vi "ConfigureMeasurementParameters.vi"(0 "NI-DMM in":refnum<class "NI-DMM.lvclass">, 5 "Configure_Parameters":variant, 11 "error in (no error)":errorcluster) -> (4 "NI-DMM out":refnum<class "NI-DMM.lvclass">, 15 "error out":errorcluster)   [LabVIEW 2020, in "Abstract_Instrument.lvlib" / "NI-DMM.lvclass"]
uses:
  NI-DMM.lvclass
  TypeDef/Configure_Parameters.ctl
  <instrlib>/niDMM/nidmm.llb/niDMM Resolution in Digits.ctl
  <instrlib>/niDMM/nidmm.llb/niDMM Configure Measurement Digits.vi
  <vilib>/MeasurementLink/MeasurementLink niDMM/MeasurementLink niDMM.lvlib
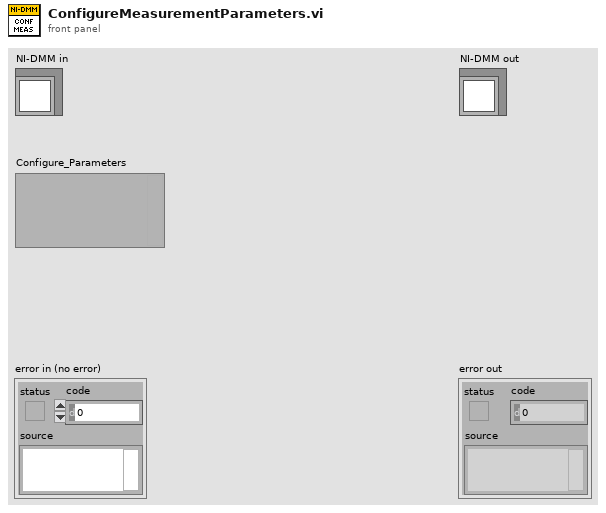
[diagram p1: front panel]
types:
  T1 = typedef "Abstract_Instrument.lvlib/NI-DMM.lvclass/Configure_Parameters.ctl" = cluster{"Range":dbl, "Measurement Type":enum32{"DC Volts", "AC Volts", "DC Current", "AC Current", "2-wire Resistance", "4-wire Resistance", "Diode", "Frequency", "Period", "AC Volts DC Coupled", "Capacitance", "Inductance", "Temperature"}, "Resolution in Digits":enum32{"3 1/2", "4 1/2", "5 1/2", "6 1/2", "7 1/2"}, "pin or relay names":string[]}
  T2 = enum32{"3 1/2", "4 1/2", "5 1/2", "6 1/2", "7 1/2"}
  T3 = enum32{"DC Volts", "AC Volts", "DC Current", "AC Current", "2-wire Resistance", "4-wire Resistance", "Diode", "Frequency", "Period", "AC Volts DC Coupled", "Capacitance", "Inductance", "Temperature"}
  T4 = typedef "MeasurementLink niDMM.lvlib/Connection with Session.ctl" = cluster{"connection":T5, "session":refnum<k15>}
  T5 = typedef "MeasurementLink Session Management V1.lvlib/Session Reservation.lvclass/Connection.ctl" = cluster{"pin or relay name":string, "site":i32, "instrument type id":string, "channel":string}
  T6 = typedef "niDMM Resolution in Digits.ctl" = dbl
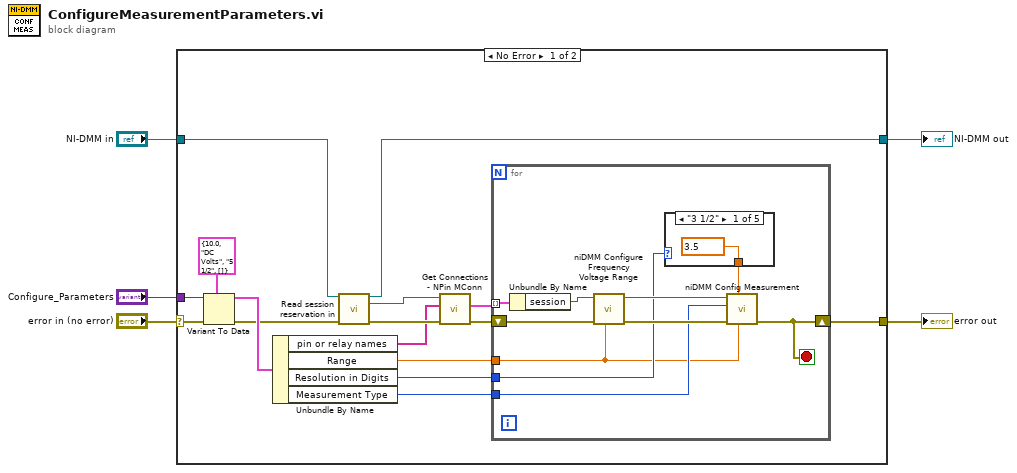
[diagram p0: block diagram]
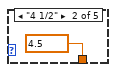
[diagram p2: hidden frame]
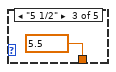
[diagram p3: hidden frame]
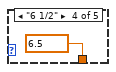
[diagram p4: hidden frame]
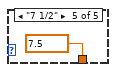
[diagram p5: hidden frame]
diagram:
  n1 = case shown="No Error" "error in (no error)" {
    selector: "error in (no error)" -> [w21 w37]
    tunnel: "NI-DMM in" -> [w12 w38]
    tunnel: "Configure_Parameters" -> [w20 _]
    tunnel: [w17 w37] -> w2
    tunnel: [w11 w38] -> w1
    frame No Error {
      n2 = Variant To Data(error in=w21, type=T1 {"Range"=10.0, "Measurement Type"=enum."DC Volts", "Resolution in Digits"=enum."5 1/2", "pin or relay names"=[]} ("Configure_Parameters"), Variant=w20) -> (data=w18:T1, error out=w13:errorcluster)
      n3 = Unbundle By Name(w18) -> ("pin or relay names"=w6:string[], "Range"=w14:dbl, "Resolution in Digits"=w15:T2, "Measurement Type"=w16:T3)
      n4 = call-dynamic "Read session reservation in.vi"("AbstractDMM in"=w12, "error in (no error)"=w13) -> ("AbstractDMM out"=w11:refnum<class "NI-DMM.lvclass">, "MeasurementLink Session Management V1.lvlib:Session Reservation.lvclass"=w10:refnum<class "Session Reservation.lvclass">, "error out"=w9:errorcluster)  [unwired: 11 in]
      n5 = call <vilib>:"Get Connections - NPin MConn.vi"("error in"=w9, "pin or relay names"=w6, "session reservation in"=w10) -> ("error out"=w8:errorcluster, "connections"=w7:T4[])  [unwired: 6 in, 1 out]
      n6 = for {
        tunnel: w16 -> [w28]
        tunnel: w15 -> [w27]
        tunnel: w14 -> [w26]
        shift-right: [w22] -> w17
        shift-left: w8 -> [w25]
        tunnel: w7 -> [w24] mode=indexing
        stop <- w22 stop-if-true
        n7 = Unbundle By Name(w24) -> ("session"=w23:refnum<k15>)
        n8 = call <instrlib>:"niDMM Configure Frequency Voltage Range.vi"("Frequency Voltage Range"=w26, "error in (no error)"=w25, "instrument handle"=w23) -> ("error out"=w31:errorcluster, "instrument handle out"=w30:refnum<k15>)  [unwired: 7 in]
        n9 = case shown="\"3 1/2\"" w27 {
          tunnel: [w32 w33 w34 w35 w36] -> w29
          frame "3 1/2" {
            w32 = T6 3.5 items=["3 1/2"=3.5, "4 1/2"=4.5, "5 1/2"=5.5, "6 1/2"=6.5, "7 1/2"=7.5] ("Resolution in Digits")
          }
          frame "4 1/2" {
            w33 = T6 4.5 items=["3 1/2"=3.5, "4 1/2"=4.5, "5 1/2"=5.5, "6 1/2"=6.5, "7 1/2"=7.5] ("Resolution in Digits")
          }
          frame "5 1/2" {
            w34 = T6 5.5 items=["3 1/2"=3.5, "4 1/2"=4.5, "5 1/2"=5.5, "6 1/2"=6.5, "7 1/2"=7.5] ("Resolution in Digits")
          }
          frame "6 1/2" {
            w35 = T6 6.5 items=["3 1/2"=3.5, "4 1/2"=4.5, "5 1/2"=5.5, "6 1/2"=6.5, "7 1/2"=7.5] ("Resolution in Digits")
          }
          frame "7 1/2" {
            w36 = T6 7.5 items=["3 1/2"=3.5, "4 1/2"=4.5, "5 1/2"=5.5, "6 1/2"=6.5, "7 1/2"=7.5] ("Resolution in Digits")
          }
        }
        n10 = call-poly <instrlib>:"niDMM Config Measurement.vi"("Range"=w26, "Resolution in Digits"=w29, "error in (no error)"=w31, "Function"=w28, "instrument handle"=w30) -> ("error out"=w22:errorcluster)  [unwired: 5 in, 1 out]
      }
    }
    frame Error {
    }
  }
  "error out" <- w2
  "NI-DMM out" <- w1
